vi "perfer straight heading.vi"(10 "min obstacle dist":u16) -> (0 "driveable paths?":bool, 3 "wheel angle":i8)   [LabVIEW 2009]
uses:
  drivable paths global.vi
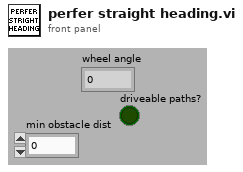
[diagram p1: front panel]
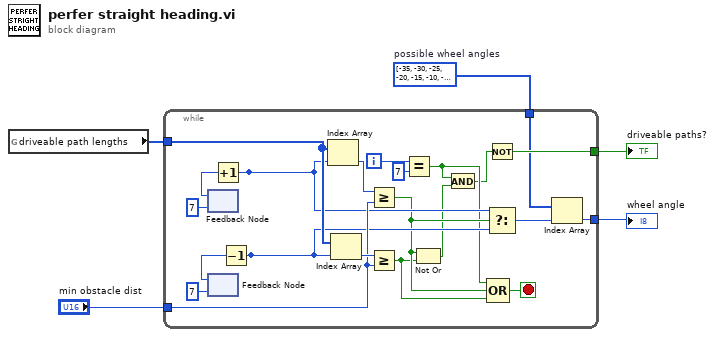
[diagram p0: block diagram]
diagram:
  w1 = i8[] [-35, -30, -25, -20, -15, -10, -5, -1, 1, 5, 10, 15, 20, 25, 30, 35]  # possible wheel angles
  n1 = global read "drivable paths global.vi" "driveable path lengths"() -> (w4:u16[])
  n2 = while {
    tunnel: w4 -> [w27]
    tunnel: "min obstacle dist" -> [w24]
    tunnel: [w19] -> w3
    tunnel: [w18] -> w2
    tunnel: w1 -> [w17]
    i -> [w23]
    stop <- w21 stop-if-true
    n3 = feedback #1(i8 7) -> (w14:i8)
    n4 = feedback #2(i8 7) -> (w12:i8)
    n5 = Increment(x=w14) -> (x+1=w16:i8)
    n6 = Decrement(x=w12) -> (x-1=w11:i8)
    n7 = Index Array(array=w27, index=w16) -> (element=w25:u16)
    n8 = Index Array(array=w27, index=w11) -> (element=w26:u16)
    n9 = Greater Or Equal?(x=w25, y=w24) -> (x >= y?=w10:bool)
    n10 = Greater Or Equal?(x=w26, y=w24) -> (x >= y?=w9:bool)
    n11 = Equal?(x=w23, y=7) -> (x = y?=w7:bool)
    n12 = Not Or(1:w9, 2:w10) -> (0:w8:bool)
    n13 = And(x=w7, y=w8) -> (x .and. y?=w6:bool)
    n14 = Not(x=w6) -> (.not. x?=w19:bool)
    n15 = Select(t=w16, s=w10, f=w11) -> (s? t:f=w20:i8)
    n16 = Compound Arithmetic op=OR(w7, w10, w9) -> (w21:bool)
    n17 = Index Array(array=w17, index=w20) -> (element=w18:i8)
  }
  "wheel angle" <- w2
  "driveable paths?" <- w3
